vi "UTIL_5PtCalibrateSave.vi"(9 "Level Raw Refnum":refnum<vi>, 10 "Input":string="LabVIEW", 11 "Sequence":i32) -> (0 "T button?":bool)   [LabVIEW 2024]
panel:
  out "Cal_Low_Laser_Reading 2":string="       2"
  out "Cal_Low_Oil_Level 2":string="       1"
  out "Cal_High_Oil_Level 2":string="       3"
  out "Cal_High_Laser_Reading  2":string="       4"
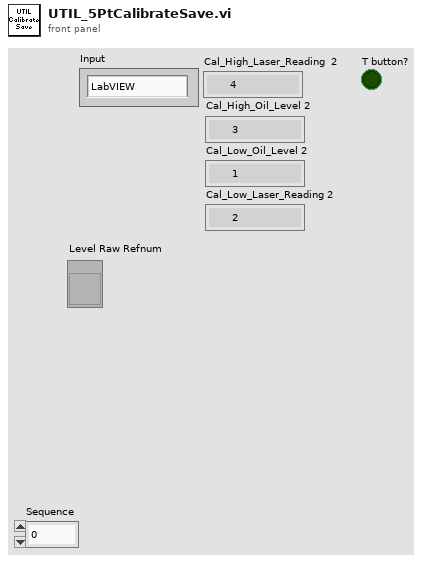
[diagram p1: front panel]
types:
  T1 = typedef "DEF_CalConstants.ctl" = cluster{"Measure High":string, "Laser High":string, "Measure Low":string, "Laser Low":string, "Cal Name":string, "Cal Date":string, "Empty Inches":dbl, "Full Inches":dbl, "Valid":bool}
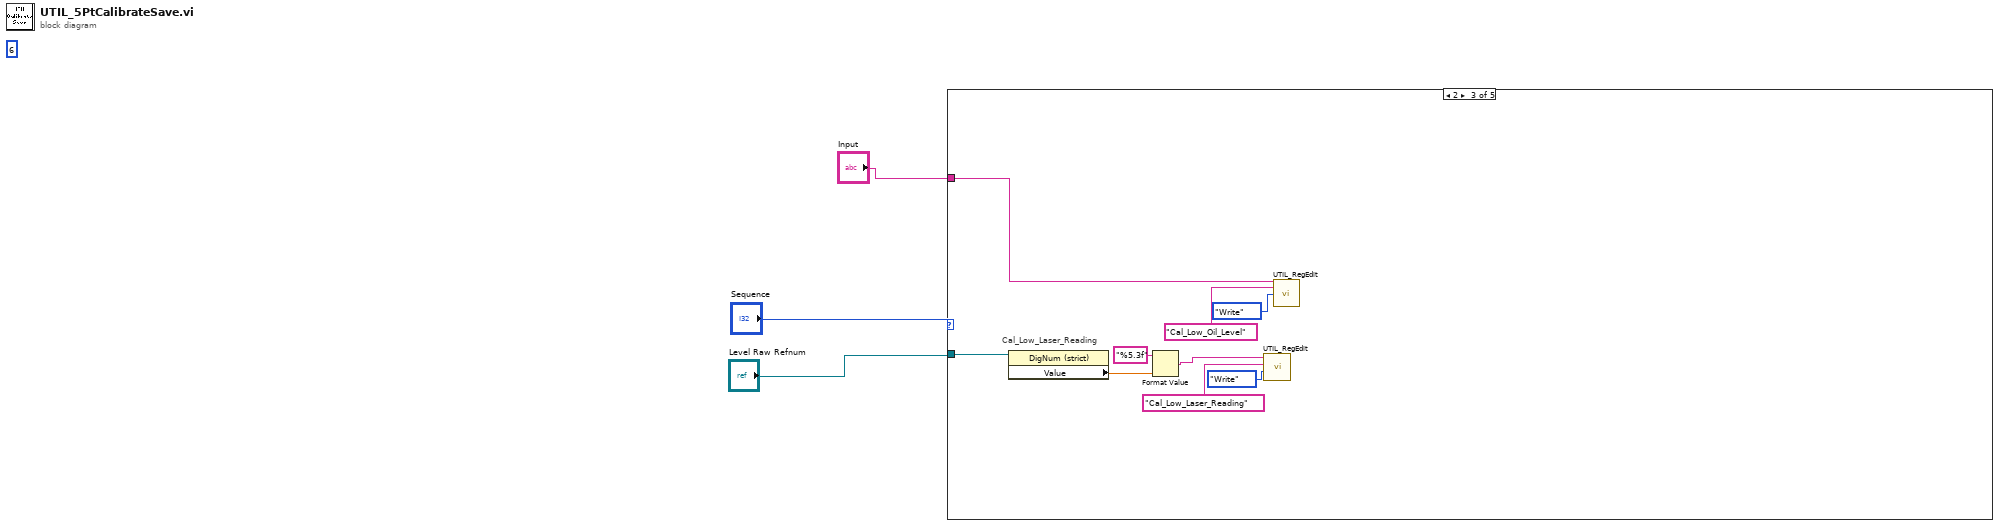
[diagram p0: block diagram]
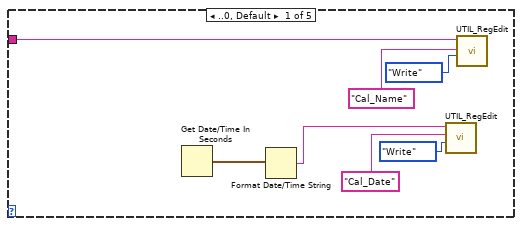
[diagram p2: hidden frame]
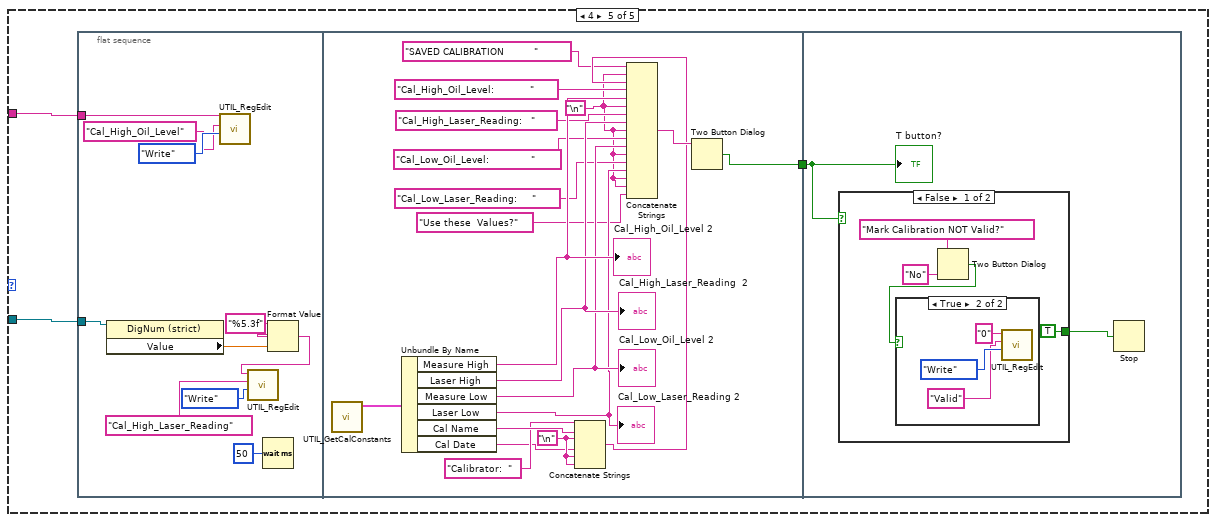
[diagram p5: hidden frame]
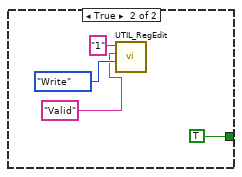
[diagram p7: hidden frame]
diagram:
  (unwired) 6
  n1 = case shown="2" "Sequence" {
    tunnel: "Level Raw Refnum" -> [_ _ w13 _ w22]
    tunnel: "Input" -> [w4 _ w11 _ w21]
    frame ..0, Default {
      n2 = Get Date/Time In Seconds() -> (seconds since 1Jan1904=w10:timestamp)
      n3 = Format Date/Time String(seconds (now)=w10) -> (date/time string=w5:string)  [unwired: 2 in]
      n4 = call "UTIL_RegEdit.vi"("Mode"=enum16{"Write", "Read", "Delete"}."Write", "String Name"="Cal_Date", "String Value"=w5) -> ()  [unwired: 7 in, 2 out]
      n5 = call "UTIL_RegEdit.vi"("Mode"=enum16{"Write", "Read", "Delete"}."Write", "String Name"="Cal_Name", "String Value"=w4) -> ()  [unwired: 7 in, 2 out]
    }
    frame 1 {
    }
    frame 2 {
      # "Cal_Low_Laser_Reading"
      n6 = property class="DigNum (strict)"(reference=w13) -> ("Value"=w12:dbl)  [unwired: 1 in, 2 out]
      n7 = Format Value(format string="%5.3f", value (0)=w12) -> (output string=w15:string)  [unwired: 1 in]
      n8 = call "UTIL_RegEdit.vi"("Mode"=enum16{"Write", "Read", "Delete"}."Write", "String Name"="Cal_Low_Laser_Reading", "String Value"=w15) -> ()  [unwired: 7 in, 2 out]
      n9 = call "UTIL_RegEdit.vi"("Mode"=enum16{"Write", "Read", "Delete"}."Write", "String Name"="Cal_Low_Oil_Level", "String Value"=w11) -> ()  [unwired: 7 in, 2 out]
    }
    frame 3 {
    }
    frame 4 {
      n10 = flat-sequence {
        tunnel: w22 -> [w30]
        tunnel: w21 -> [w26]
        tunnel: [w33] -> w20
        tunnel: w20 -> [w53]
        frame #0 {
          n11 = property class="DigNum (strict)"(reference=w30) -> ("Value"=w32:dbl)  [unwired: 1 in, 2 out]
          n12 = call "UTIL_RegEdit.vi"("Mode"=enum16{"Write", "Read", "Delete"}."Write", "String Name"="Cal_High_Oil_Level", "String Value"=w26) -> ()  [unwired: 7 in, 2 out]
          n13 = Wait (ms)(milliseconds to wait=u32 50) -> ()  [unwired: 1 out]
          n14 = Format Value(format string="%5.3f", value (0)=w32) -> (output string=w31:string)  [unwired: 1 in]
          n15 = call "UTIL_RegEdit.vi"("Mode"=enum16{"Write", "Read", "Delete"}."Write", "String Name"="Cal_High_Laser_Reading", "String Value"=w31) -> ()  [unwired: 7 in, 2 out]
        }
        frame #1 {
          w36 = "\n"
          w38 = "\n"
          n16 = call "UTIL_GetCalConstants.vi"() -> ("Cal Constants"=w34:T1)  [unwired: 10 in, 1 out]
          n17 = Unbundle By Name(w34) -> ("Measure High"=w50:string, "Laser High"=w48:string, "Measure Low"=w46:string, "Laser Low"=w44:string, "Cal Name"=w41:string, "Cal Date"=w35:string)
          "Cal_High_Laser_Reading  2" <- w48
          "Cal_High_Oil_Level 2" <- w50
          "Cal_Low_Oil_Level 2" <- w46
          "Cal_Low_Laser_Reading 2" <- w44
          n18 = Concatenate Strings("Calibrator:  " ("string"), w41, w36, w35, w36, w36) -> (w40:string)
          n19 = Concatenate Strings("SAVED CALIBRATION          ", w38, w40, "Cal_High_Oil_Level:            ", w50, w38, "Cal_High_Laser_Reading:   ", w48, w38, "Cal_Low_Oil_Level:              ", w46, w38, "Cal_Low_Laser_Reading:     ", w44, w38, w38, "Use these  Values?" ("message")) -> (w42:string)
          n20 = Two Button Dialog(message=w42) -> (T button?=w33:bool)  [unwired: 2 in]
        }
        frame #2 {
          n21 = case shown="False" w53 {
            tunnel: [TRUE ("stop? (T)") TRUE ("stop? (T)")] -> w52
            frame False {
              n22 = Two Button Dialog(message="Mark Calibration NOT Valid?", 1:"No" ("F button name (\"Cancel\")")) -> (T button?=w57:bool)  [unwired: 1 in]
              n23 = case shown="True" w57 {
                frame False {
                }
                frame True {
                  n24 = call "UTIL_RegEdit.vi"("Mode"=enum16{"Write", "Read", "Delete"}."Write", "String Name"="Valid", "String Value"="0") -> ()  [unwired: 7 in, 2 out]
                }
              }
            }
            frame True {
              n25 = call "UTIL_RegEdit.vi"("Mode"=enum16{"Write", "Read", "Delete"}."Write", "String Name"="Valid", "String Value"="1") -> ()  [unwired: 7 in, 2 out]
            }
          }
          n26 = Stop(stop? (T)=w52) -> ()
          "T button?" <- w53
        }
      }
    }
  }
